vi "OdometricNavigation.vi"(0 "Wheel Angles (rad)":T3 {"RR Angle (rad)" scale=3.1416..-3.1416; "RL Angle (rad)" scale=3.1416..-3.1416; "FR Angle (rad)" scale=3.1416..-3.1416; "FL Angle (rad)" scale=3.1416..-3.1416}, 1 "Wheel Movements (in.)":cluster{"FL":dbl, "FR":dbl, "RL":dbl, "RR":dbl} {"RR" scale=-70.0..70.0; "RL" scale=-70.0..70.0; "FR" scale=-70.0..70.0; "FL" scale=-70.0..70.0}, 2 "Robot angle (degrees)":dbl(knob) scale=180.0..-180.0, 3 "x and y error minimum (in.)":dbl, 4 "error minimum for rotation (rad)":dbl) -> (17 "movement":cluster{"sy":dbl, "sx":dbl, "rot.":dbl})   [LabVIEW 2015, in "Team900SwerveDrive.lvlib"]
uses:
  Team900SwerveDrive.lvlib
  <vilib>/Analysis/baseanly.llb/Mean (DBL).vi
  SwerveGlobalData.vi
  <vilib>/Analysis/NI_AALBase.lvlib
panel:
  out "unhandled error data":dbl[][](array[numeric])
  out "Wheel X movements":T1
  out "Wheel Y movements":T2
  out "1-side error rotation (rad)":dbl
  out "compared":cluster{"sy":dbl, "sx":dbl, "rot.":dbl}[](array[cluster])
  out "Right Error":bool
  out "Front Error":bool
  out "Rear Error":bool
  out "Left Error":bool
  # "This VI should be run in periodic tasks at about 10 Hz, with the results being added to the\nX and Y elements of the 'Coordinates' variable from SwerveGlobalData.vi. Requires inputs of\ndelta(position) in inches and angle in radians for each wheel, as well as robot angle (in degrees)\nand error tolerances for the delta(position) and delta(angle) of the robot.\n\nThought: separate the X and Y coordinates of the robot and the heading of the robot into\ntwo separate global variables.\n\nThought: standardize degrees or radians throughout the code. Currently radians are used for\neverything except robot heading."
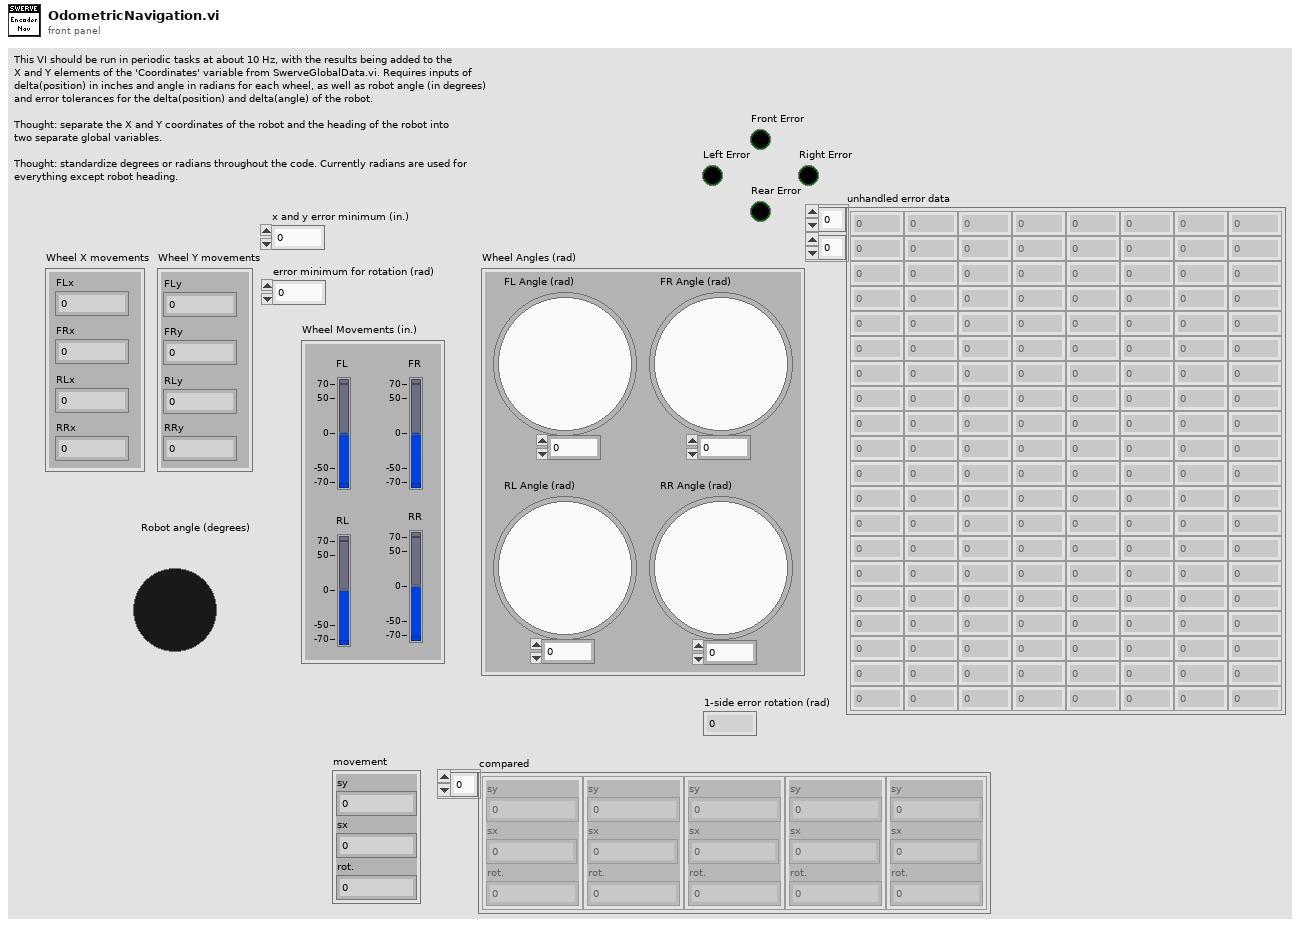
[diagram p1: front panel]
types:
  T1 = cluster{"FLx":dbl, "FRx":dbl, "RLx":dbl, "RRx":dbl}
  T2 = cluster{"FLy":dbl, "FRy":dbl, "RLy":dbl, "RRy":dbl}
  T3 = cluster{"FL Angle (rad)":dbl, "FR Angle (rad)":dbl, "RL Angle (rad)":dbl, "RR Angle (rad)":dbl}
  T4 = cluster{"[0]":dbl, "[1]":dbl, "[2]":dbl, "[3]":dbl}
  T5 = enum16{"no error", "front", "rear", "left", "right", "FL", "FR", "RL", "RR", "other"}
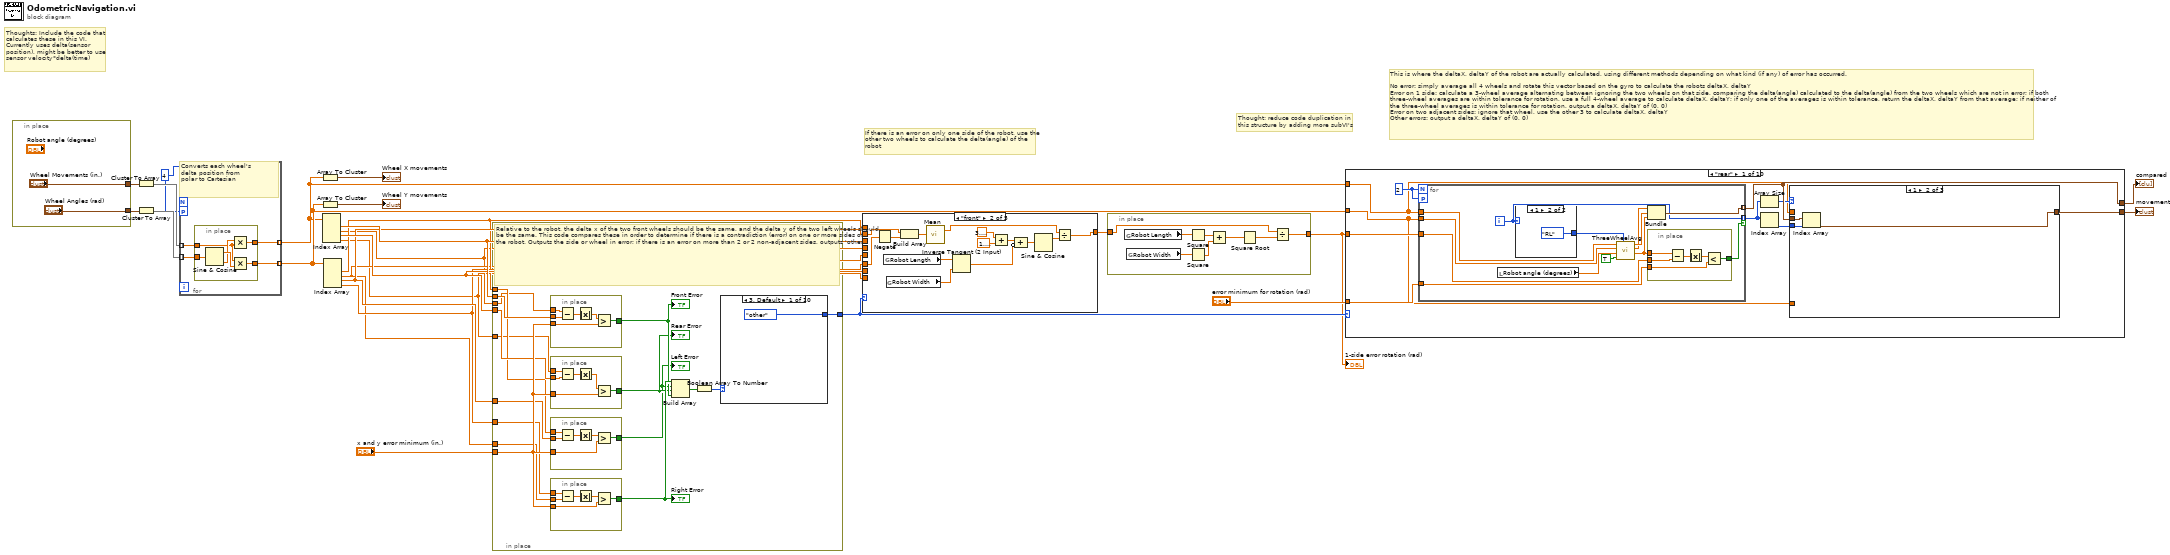
[diagram p0: block diagram]
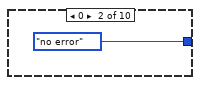
[diagram p2: hidden frame]
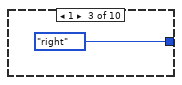
[diagram p3: hidden frame]
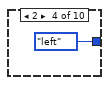
[diagram p4: hidden frame]
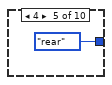
[diagram p5: hidden frame]
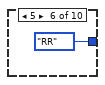
[diagram p6: hidden frame]
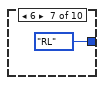
[diagram p7: hidden frame]
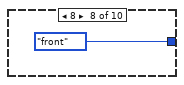
[diagram p8: hidden frame]
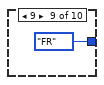
[diagram p9: hidden frame]
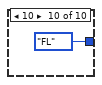
[diagram p10: hidden frame]
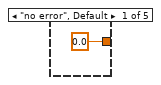
[diagram p11: hidden frame]
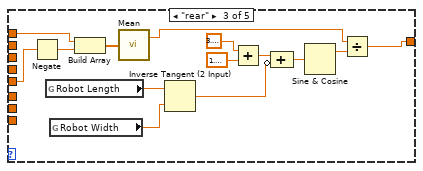
[diagram p12: hidden frame]
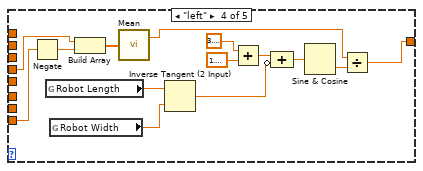
[diagram p13: hidden frame]
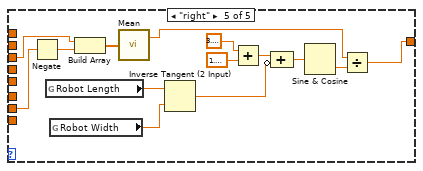
[diagram p14: hidden frame]
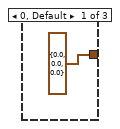
[diagram p15: hidden frame]
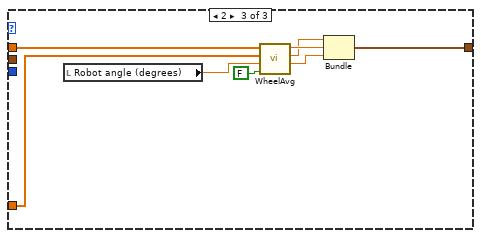
[diagram p16: hidden frame]
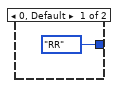
[diagram p17: hidden frame]
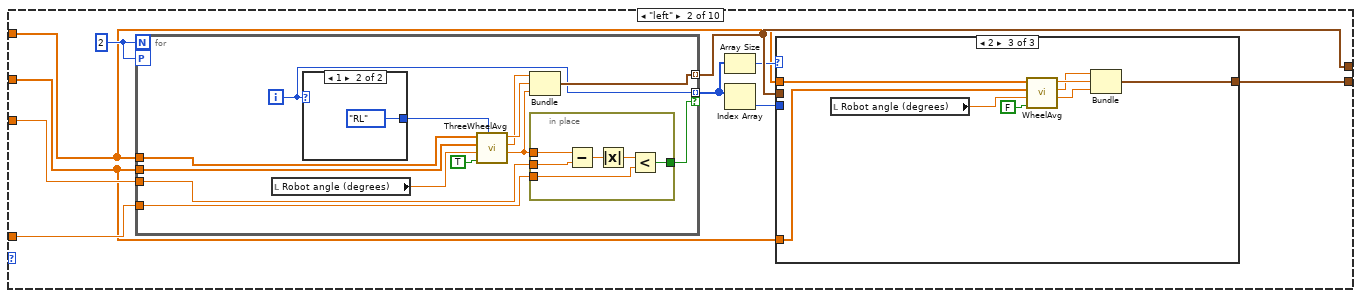
[diagram p18: hidden frame]
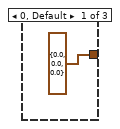
[diagram p19: hidden frame]
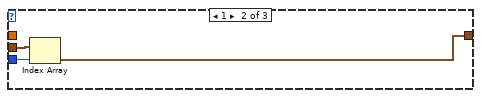
[diagram p20: hidden frame]
diagram:
  w16 = 4
  # "Thought: reduce code duplication in\nthis structure by adding more subVI's"
  # "This is where the deltaX, deltaY of the robot are actually calculated, using different methods depending on what kind (if any) of error has occurred.\n\nNo error: simply average all 4 wheels and rotate this vector based on the gyro to calculate the robots deltaX, deltaY\nError on 1 side: calculate a 3-wheel average alternating between ignoring the two wheels on that side, comparing the delta(angle) calculated to the delta(angle) from the two wheels which are not in error; if both \nthree-wheel averages are within tolerance for rotation, use a full 4-wheel average to calculate deltaX, deltaY; if only one of the averages is within tolerance, return the deltaX, deltaY from that average; if neither of\nthe three-wheel averages is within tolerance for rotation, output a deltaX, deltaY of (0, 0)\nError on two adjacent sides: ignore that wheel, use the other 3 to calculate deltaX, deltaY\nOther errors: output a deltaX, deltaY of (0, 0)"
  # "If there is an error on only one side of the robot, use the\nother two wheels to calculate the delta(angle) of the\nrobot"
  # "Thoughts: Include the code that\ncalculates these in this VI. \nCurrently uses delta(sensor\nposition), might be better to use\nsensor velocity*delta(time)"
  n1 = in-place {
    in-place-border: ["Wheel Movements (in.)"] -> w19
    in-place-border: ["Wheel Angles (rad)"] -> w18
  }
  n2 = Cluster To Array(cluster=w19) -> (array=w20:dbl[])
  n3 = Cluster To Array(cluster=w18) -> (array=w17:dbl[])
  n4 = for {
    N: w16 -> [_]
    tunnel: w20 -> [w30] mode=indexing
    tunnel: w17 -> [w29] mode=indexing
    workers-P: w16 -> [_]
    tunnel: [w28] -> w3 mode=indexing
    tunnel: [w27] -> w2 mode=indexing
    # "Converts each wheel's\ndelta position from\npolar to Cartesian"
    n5 = in-place {
      in-place-border: [w34] -> w27
      in-place-border: [w33] -> w28
      in-place-border: w30 -> [w32]
      in-place-border: w29 -> [w31]
      n6 = Sine & Cosine(0:w31) -> (1:w36:dbl, 2:w35:dbl)
      n7 = Multiply(x=w35, y=w32) -> (x*y=w34:dbl)
      n8 = Multiply(x=w32, y=w36) -> (x*y=w33:dbl)
    }
  }
  n9 = Array To Cluster(array=w2) -> (cluster=→"Wheel X movements":T4)
  n10 = Array To Cluster(array=w3) -> (cluster=→"Wheel Y movements":T4)
  n11 = Index Array(array=w2) -> (element #1=w12:dbl, element #2=w6:dbl, element #3=w11:dbl, element #4=w5:dbl)  [unwired: 4 in]
  n12 = Index Array(array=w3) -> (element #1=w8:dbl, element #2=w7:dbl, element #3=w10:dbl, element #4=w9:dbl)  [unwired: 4 in]
  n13 = in-place {
    in-place-border: "x and y error minimum (in.)" -> [w52]
    in-place-border: [w45] -> w13
    in-place-border: w12 -> [w44]
    in-place-border: w11 -> [w43]
    in-place-border: w10 -> [w42]
    in-place-border: w9 -> [w41]
    in-place-border: w8 -> [w40]
    in-place-border: w7 -> [w39]
    in-place-border: w6 -> [w38]
    in-place-border: w5 -> [w37]
    # "Relative to the robot, the delta x of the two front wheels should be the same, and the delta y of the two left wheels should be the same. This code compares these in order to determine if there is a contradiction (error) on one or more sides of the robot. Outputs the side or wheel in error; if there is an error on more than 2 or 2 non-adjacent sides, outputs 'other.'"
    n14 = in-place {
      in-place-border: [w66] -> w48
      in-place-border: w38 -> [w65]
      in-place-border: w44 -> [w64]
      in-place-border: w52 -> [w63]
      n15 = Subtract(x=w65, y=w64) -> (x-y=w68:dbl)
      n16 = Absolute Value(x=w68) -> (abs(x)=w67:dbl)
      n17 = Greater?(x=w67, y=w63) -> (0:w66:bool)
    }
    "Front Error" <- w48
    n18 = in-place {
      in-place-border: [w72] -> w47
      in-place-border: w37 -> [w71]
      in-place-border: w43 -> [w70]
      in-place-border: w52 -> [w69]
      n19 = Subtract(x=w71, y=w70) -> (x-y=w74:dbl)
      n20 = Absolute Value(x=w74) -> (abs(x)=w73:dbl)
      n21 = Greater?(x=w73, y=w69) -> (0:w72:bool)
    }
    "Rear Error" <- w47
    n22 = in-place {
      in-place-border: [w78] -> w46
      in-place-border: w40 -> [w77]
      in-place-border: w42 -> [w76]
      in-place-border: w52 -> [w75]
      n23 = Subtract(x=w77, y=w76) -> (x-y=w80:dbl)
      n24 = Absolute Value(x=w80) -> (abs(x)=w79:dbl)
      n25 = Greater?(x=w79, y=w75) -> (0:w78:bool)
    }
    "Left Error" <- w46
    n26 = in-place {
      in-place-border: [w84] -> w49
      in-place-border: w41 -> [w83]
      in-place-border: w39 -> [w82]
      in-place-border: w52 -> [w81]
      n27 = Subtract(x=w83, y=w82) -> (x-y=w86:dbl)
      n28 = Absolute Value(x=w86) -> (abs(x)=w85:dbl)
      n29 = Greater?(x=w85, y=w81) -> (0:w84:bool)
    }
    "Right Error" <- w49
    n30 = Build Array(w49, w46, w47, w48) -> (w51:bool[])
    n31 = Boolean Array To Number(Boolean array=w51) -> (number=w50:u32)
    n32 = case shown="3, Default" w50 {
      tunnel: [T5."other" T5."no error" T5."right" T5."left" T5."rear" T5."RR" T5."RL" T5."front" T5."FR" T5."FL"] -> w45
      frame 3, Default {
      }
      frame 0 {
      }
      frame 1 {
      }
      frame 2 {
      }
      frame 4 {
      }
      frame 5 {
      }
      frame 6 {
      }
      frame 8 {
      }
      frame 9 {
      }
      frame 10 {
      }
    }
  }
  n33 = case shown="\"front\"" w13 {
    tunnel: [0.0 w90 w102 w116 w132] -> w4
    tunnel: w12 -> [_ _ _ _ w131]
    tunnel: w11 -> [_ _ _ _ w130]
    tunnel: w10 -> [_ w89 _ _ _]
    tunnel: w9 -> [_ w88 _ _ _]
    tunnel: w8 -> [_ _ w105 _ _]
    tunnel: w7 -> [_ _ w104 _ _]
    tunnel: w6 -> [_ _ _ w118 _]
    tunnel: w5 -> [_ _ _ w117 _]
    frame "no error", Default {
    }
    frame "front" {
      n34 = Negate(x=w88) -> (-x=w100:dbl)
      n35 = global read "SwerveGlobalData.vi" "Robot Length"() -> (w93:dbl)
      n36 = global read "SwerveGlobalData.vi" "Robot Width"() -> (w94:dbl)
      n37 = Build Array(w89, w100) -> (w101:dbl[])
      n38 = call-poly <vilib>:"Mean.vi"("X"=w101) -> ("mean"=w99:dbl)  [unwired: 1 out]
      n39 = Inverse Tangent (2 Input)(1:w94, 2:w93) -> (0:w95:dbl)
      n40 = Add(x=3.141592653589793, y=1.5707963267948966) -> (x+y=w96:dbl)
      n41 = Compound Arithmetic op=ADD(w96, invert w95) -> (w92:dbl)
      n42 = Sine & Cosine(0:w92) -> (1:w91:dbl)  [unwired: 1 out]
      n43 = Divide(x=w99, y=w91) -> (x/y=w90:dbl)
    }
    frame "rear" {
      n44 = Negate(x=w104) -> (-x=w114:dbl)
      n45 = global read "SwerveGlobalData.vi" "Robot Length"() -> (w108:dbl)
      n46 = global read "SwerveGlobalData.vi" "Robot Width"() -> (w109:dbl)
      n47 = Build Array(w105, w114) -> (w115:dbl[])
      n48 = call-poly <vilib>:"Mean.vi"("X"=w115) -> ("mean"=w113:dbl)  [unwired: 1 out]
      n49 = Inverse Tangent (2 Input)(1:w109, 2:w108) -> (0:w103:dbl)
      n50 = Add(x=3.141592653589793, y=1.5707963267948966) -> (x+y=w110:dbl)
      n51 = Compound Arithmetic op=ADD(w110, invert w103) -> (w107:dbl)
      n52 = Sine & Cosine(0:w107) -> (1:w106:dbl)  [unwired: 1 out]
      n53 = Divide(x=w113, y=w106) -> (x/y=w102:dbl)
    }
    frame "left" {
      n54 = Negate(x=w117) -> (-x=w128:dbl)
      n55 = global read "SwerveGlobalData.vi" "Robot Length"() -> (w121:dbl)
      n56 = global read "SwerveGlobalData.vi" "Robot Width"() -> (w122:dbl)
      n57 = Build Array(w118, w128) -> (w129:dbl[])
      n58 = call-poly <vilib>:"Mean.vi"("X"=w129) -> ("mean"=w127:dbl)  [unwired: 1 out]
      n59 = Inverse Tangent (2 Input)(1:w122, 2:w121) -> (0:w123:dbl)
      n60 = Add(x=3.141592653589793, y=1.5707963267948966) -> (x+y=w124:dbl)
      n61 = Compound Arithmetic op=ADD(w124, invert w123) -> (w120:dbl)
      n62 = Sine & Cosine(0:w120) -> (2:w119:dbl)  [unwired: 1 out]
      n63 = Divide(x=w127, y=w119) -> (x/y=w116:dbl)
    }
    frame "right" {
      n64 = Negate(x=w130) -> (-x=w142:dbl)
      n65 = global read "SwerveGlobalData.vi" "Robot Length"() -> (w136:dbl)
      n66 = global read "SwerveGlobalData.vi" "Robot Width"() -> (w137:dbl)
      n67 = Build Array(w131, w142) -> (w143:dbl[])
      n68 = call-poly <vilib>:"Mean.vi"("X"=w143) -> ("mean"=w134:dbl)  [unwired: 1 out]
      n69 = Inverse Tangent (2 Input)(1:w137, 2:w136) -> (0:w138:dbl)
      n70 = Add(x=3.141592653589793, y=1.5707963267948966) -> (x+y=w139:dbl)
      n71 = Compound Arithmetic op=ADD(w139, invert w138) -> (w135:dbl)
      n72 = Sine & Cosine(0:w135) -> (2:w133:dbl)  [unwired: 1 out]
      n73 = Divide(x=w134, y=w133) -> (x/y=w132:dbl)
    }
  }
  n74 = in-place {
    in-place-border: w4 -> [w145]
    in-place-border: [w144] -> w1
    n75 = global read "SwerveGlobalData.vi" "Robot Length"() -> (w151:dbl)
    n76 = global read "SwerveGlobalData.vi" "Robot Width"() -> (w150:dbl)
    n77 = Square(x=w151) -> (x^2=w148:dbl)
    n78 = Square(x=w150) -> (x^2=w149:dbl)
    n79 = Add(x=w148, y=w149) -> (x+y=w147:dbl)
    n80 = Square Root(x=w147) -> (sqrt(x)=w146:dbl)
    n81 = Divide(x=w145, y=w146) -> (x/y=w144:dbl)
  }
  "1-side error rotation (rad)" <- w1
  n82 = case shown="\"rear\"" w13 {
    tunnel: [w157 w200 w243 w286 cluster{"mean":dbl, "mean":dbl, "mean":dbl}[] [] cluster{"mean":dbl, "mean":dbl, "mean":dbl}[] [] cluster{"mean":dbl, "mean":dbl, "mean":dbl}[] [] cluster{"mean":dbl, "mean":dbl, "mean":dbl}[] [] cluster{"mean":dbl, "mean":dbl, "mean":dbl}[] [] cluster{"mean":dbl, "mean":dbl, "mean":dbl}[] []] -> w23
    tunnel: "error minimum for rotation (rad)" -> [w161 w204 w247 w290 _ _ _ _ _ _]
    tunnel: [w158 w201 w244 w287 w333 w343 w353 w363 cluster{"mean":dbl, "mean":dbl, "mean":dbl} {"mean"=0.0, "mean"=0.0, "mean"=0.0} w379] -> w21
    tunnel: w3 -> [w153 w196 w239 w282 w329 w339 w349 w359 w368 w374]
    tunnel: w2 -> [w152 w195 w238 w281 w328 w338 w348 w358 w369 w373]
    tunnel: w1 -> [w156 w199 w242 w285 _ _ _ _ _ _]
    frame "rear" {
      w155 = 2
      n83 = for {
        N: w155 -> [_]
        tunnel: [w186] -> w157 mode=indexing
        tunnel: w161 -> [w185]
        tunnel: [w184] -> w160 mode=indexing if=w183
        tunnel: w153 -> [w180]
        tunnel: w152 -> [w179]
        tunnel: w156 -> [w174]
        workers-P: w155 -> [_]
        i -> [w184]
        n84 = local read "Robot angle (degrees)"() -> (w181:dbl)
        n85 = case shown="1" w184 {
          tunnel: [enum16{"FL", "FR", "RL", "RR"}."RR" ("Wheel Missing") enum16{"FL", "FR", "RL", "RR"}."RL" ("Wheel Missing")] -> w178
          frame 0, Default {
          }
          frame 1 {
          }
        }
        n86 = call "ThreeWheelAvg.vi"("Wheel Missing"=w178, "Calculate Rotation?"=TRUE, "Robot Angle (degrees)"=w181, "wheel Y movements (FL, FR, RL, RR)"=w180, "wheel X movements (FL, FR, RL, RR)"=w179) -> ("Rotation"=w175:dbl, "Y"=w176:dbl, "X"=w177:dbl)  [unwired: 4 in]
        n87 = Bundle("Y"=w176, "X"=w177, "Rotation"=w175) -> (w186:cluster{"Y":dbl, "X":dbl, "Rotation":dbl})  [unwired: 1 in]
        n88 = in-place {
          in-place-border: [w190] -> w183
          in-place-border: w185 -> [w189]
          in-place-border: w175 -> [w188]
          in-place-border: w174 -> [w187]
          n89 = Subtract(x=w188, y=w187) -> (x-y=w192:dbl)
          n90 = Absolute Value(x=w192) -> (abs(x)=w191:dbl)
          n91 = Less?(x=w191, y=w189) -> (x < y?=w190:bool)
        }
      }
      n92 = Array Size(array=w160) -> (size(s)=w154:i32)
      n93 = Index Array(array=w160) -> (element=w159:i32)  [unwired: 1 in]
      n94 = case shown="1" w154 {
        tunnel: w159 -> [_ w163 _]
        tunnel: [cluster{"Y":dbl, "X":dbl, "Rotation":dbl} {"Y"=0.0, "X"=0.0, "Rotation"=0.0} w165 w168] -> w158
        tunnel: w157 -> [_ w164 _]
        tunnel: w153 -> [_ _ w173]
        tunnel: w152 -> [_ _ w172]
        frame 0, Default {
        }
        frame 1 {
          n95 = Index Array(array=w164, index=w163) -> (element=w165:cluster{"Y":dbl, "X":dbl, "Rotation":dbl})
        }
        frame 2 {
          n96 = local read "Robot angle (degrees)"() -> (w166:dbl)
          n97 = call "WheelAvg.vi"("Calculate Rotation?"=FALSE, "Robot Angle (degrees)"=w166, "wheel Y movements (FL, FR, RL, RR)"=w173, "wheel X movements (FL, FR, RL, RR)"=w172) -> ("Rotation"=w169:dbl, "Y"=w170:dbl, "X"=w171:dbl)  [unwired: 5 in]
          n98 = Bundle("Y"=w170, "X"=w171, "Rotation"=w169) -> (w168:cluster{"Y":dbl, "X":dbl, "Rotation":dbl})  [unwired: 1 in]
        }
      }
    }
    frame "left" {
      w198 = 2
      n99 = for {
        N: w198 -> [_]
        tunnel: [w229] -> w200 mode=indexing
        tunnel: w204 -> [w228]
        tunnel: [w227] -> w203 mode=indexing if=w226
        tunnel: w196 -> [w223]
        tunnel: w195 -> [w222]
        tunnel: w199 -> [w217]
        workers-P: w198 -> [_]
        i -> [w227]
        n100 = local read "Robot angle (degrees)"() -> (w224:dbl)
        n101 = case shown="1" w227 {
          tunnel: [enum16{"FL", "FR", "RL", "RR"}."RR" ("Wheel Missing") enum16{"FL", "FR", "RL", "RR"}."RL" ("Wheel Missing")] -> w221
          frame 0, Default {
          }
          frame 1 {
          }
        }
        n102 = call "ThreeWheelAvg.vi"("Wheel Missing"=w221, "Calculate Rotation?"=TRUE, "Robot Angle (degrees)"=w224, "wheel Y movements (FL, FR, RL, RR)"=w223, "wheel X movements (FL, FR, RL, RR)"=w222) -> ("Rotation"=w218:dbl, "Y"=w219:dbl, "X"=w220:dbl)  [unwired: 4 in]
        n103 = Bundle("Y"=w219, "X"=w220, "Rotation"=w218) -> (w229:cluster{"Y":dbl, "X":dbl, "Rotation":dbl})  [unwired: 1 in]
        n104 = in-place {
          in-place-border: [w233] -> w226
          in-place-border: w228 -> [w232]
          in-place-border: w218 -> [w231]
          in-place-border: w217 -> [w230]
          n105 = Subtract(x=w231, y=w230) -> (x-y=w235:dbl)
          n106 = Absolute Value(x=w235) -> (abs(x)=w234:dbl)
          n107 = Less?(x=w234, y=w232) -> (x < y?=w233:bool)
        }
      }
      n108 = Array Size(array=w203) -> (size(s)=w197:i32)
      n109 = Index Array(array=w203) -> (element=w202:i32)  [unwired: 1 in]
      n110 = case shown="2" w197 {
        tunnel: w202 -> [_ w206 _]
        tunnel: [cluster{"Y":dbl, "X":dbl, "Rotation":dbl} {"Y"=0.0, "X"=0.0, "Rotation"=0.0} w208 w211] -> w201
        tunnel: w200 -> [_ w207 _]
        tunnel: w196 -> [_ _ w216]
        tunnel: w195 -> [_ _ w215]
        frame 0, Default {
        }
        frame 1 {
          n111 = Index Array(array=w207, index=w206) -> (element=w208:cluster{"Y":dbl, "X":dbl, "Rotation":dbl})
        }
        frame 2 {
          n112 = local read "Robot angle (degrees)"() -> (w209:dbl)
          n113 = call "WheelAvg.vi"("Calculate Rotation?"=FALSE, "Robot Angle (degrees)"=w209, "wheel Y movements (FL, FR, RL, RR)"=w216, "wheel X movements (FL, FR, RL, RR)"=w215) -> ("Rotation"=w212:dbl, "Y"=w213:dbl, "X"=w214:dbl)  [unwired: 5 in]
          n114 = Bundle("Y"=w213, "X"=w214, "Rotation"=w212) -> (w211:cluster{"Y":dbl, "X":dbl, "Rotation":dbl})  [unwired: 1 in]
        }
      }
    }
    frame "right" {
      w241 = 2
      n115 = for {
        N: w241 -> [_]
        tunnel: [w272] -> w243 mode=indexing
        tunnel: w247 -> [w271]
        tunnel: [w270] -> w246 mode=indexing if=w269
        tunnel: w239 -> [w266]
        tunnel: w238 -> [w265]
        tunnel: w242 -> [w260]
        workers-P: w241 -> [_]
        i -> [w270]
        n116 = local read "Robot angle (degrees)"() -> (w267:dbl)
        n117 = case shown="1" w270 {
          tunnel: [enum16{"FL", "FR", "RL", "RR"}."RR" ("Wheel Missing") enum16{"FL", "FR", "RL", "RR"}."RL" ("Wheel Missing")] -> w264
          frame 0, Default {
          }
          frame 1 {
          }
        }
        n118 = call "ThreeWheelAvg.vi"("Wheel Missing"=w264, "Calculate Rotation?"=TRUE, "Robot Angle (degrees)"=w267, "wheel Y movements (FL, FR, RL, RR)"=w266, "wheel X movements (FL, FR, RL, RR)"=w265) -> ("Rotation"=w261:dbl, "Y"=w262:dbl, "X"=w263:dbl)  [unwired: 4 in]
        n119 = Bundle("Y"=w262, "X"=w263, "Rotation"=w261) -> (w272:cluster{"Y":dbl, "X":dbl, "Rotation":dbl})  [unwired: 1 in]
        n120 = in-place {
          in-place-border: [w276] -> w269
          in-place-border: w271 -> [w275]
          in-place-border: w261 -> [w274]
          in-place-border: w260 -> [w273]
          n121 = Subtract(x=w274, y=w273) -> (x-y=w278:dbl)
          n122 = Absolute Value(x=w278) -> (abs(x)=w277:dbl)
          n123 = Less?(x=w277, y=w275) -> (x < y?=w276:bool)
        }
      }
      n124 = Array Size(array=w246) -> (size(s)=w240:i32)
      n125 = Index Array(array=w246) -> (element=w245:i32)  [unwired: 1 in]
      n126 = case shown="2" w240 {
        tunnel: w245 -> [_ w249 _]
        tunnel: [cluster{"Y":dbl, "X":dbl, "Rotation":dbl} {"Y"=0.0, "X"=0.0, "Rotation"=0.0} w251 w254] -> w244
        tunnel: w243 -> [_ w250 _]
        tunnel: w239 -> [_ _ w259]
        tunnel: w238 -> [_ _ w258]
        frame 0, Default {
        }
        frame 1 {
          n127 = Index Array(array=w250, index=w249) -> (element=w251:cluster{"Y":dbl, "X":dbl, "Rotation":dbl})
        }
        frame 2 {
          n128 = local read "Robot angle (degrees)"() -> (w252:dbl)
          n129 = call "WheelAvg.vi"("Calculate Rotation?"=FALSE, "Robot Angle (degrees)"=w252, "wheel Y movements (FL, FR, RL, RR)"=w259, "wheel X movements (FL, FR, RL, RR)"=w258) -> ("Rotation"=w255:dbl, "Y"=w256:dbl, "X"=w257:dbl)  [unwired: 5 in]
          n130 = Bundle("Y"=w256, "X"=w257, "Rotation"=w255) -> (w254:cluster{"Y":dbl, "X":dbl, "Rotation":dbl})  [unwired: 1 in]
        }
      }
    }
    frame "front" {
      w284 = 2
      n131 = for {
        N: w284 -> [_]
        tunnel: [w315] -> w286 mode=indexing
        tunnel: w290 -> [w314]
        tunnel: [w313] -> w289 mode=indexing if=w312
        tunnel: w282 -> [w309]
        tunnel: w281 -> [w308]
        tunnel: w285 -> [w303]
        workers-P: w284 -> [_]
        i -> [w313]
        n132 = local read "Robot angle (degrees)"() -> (w310:dbl)
        n133 = case shown="1" w313 {
          tunnel: [enum16{"FL", "FR", "RL", "RR"}."RR" ("Wheel Missing") enum16{"FL", "FR", "RL", "RR"}."RL" ("Wheel Missing")] -> w307
          frame 0, Default {
          }
          frame 1 {
          }
        }
        n134 = call "ThreeWheelAvg.vi"("Wheel Missing"=w307, "Calculate Rotation?"=TRUE, "Robot Angle (degrees)"=w310, "wheel Y movements (FL, FR, RL, RR)"=w309, "wheel X movements (FL, FR, RL, RR)"=w308) -> ("Rotation"=w304:dbl, "Y"=w305:dbl, "X"=w306:dbl)  [unwired: 4 in]
        n135 = Bundle("Y"=w305, "X"=w306, "Rotation"=w304) -> (w315:cluster{"Y":dbl, "X":dbl, "Rotation":dbl})  [unwired: 1 in]
        n136 = in-place {
          in-place-border: [w319] -> w312
          in-place-border: w314 -> [w318]
          in-place-border: w304 -> [w317]
          in-place-border: w303 -> [w316]
          n137 = Subtract(x=w317, y=w316) -> (x-y=w321:dbl)
          n138 = Absolute Value(x=w321) -> (abs(x)=w320:dbl)
          n139 = Less?(x=w320, y=w318) -> (x < y?=w319:bool)
        }
      }
      n140 = Array Size(array=w289) -> (size(s)=w283:i32)
      n141 = Index Array(array=w289) -> (element=w288:i32)  [unwired: 1 in]
      n142 = case shown="0, Default" w283 {
        tunnel: w288 -> [_ w292 _]
        tunnel: [cluster{"Y":dbl, "X":dbl, "Rotation":dbl} {"Y"=0.0, "X"=0.0, "Rotation"=0.0} w294 w297] -> w287
        tunnel: w286 -> [_ w293 _]
        tunnel: w282 -> [_ _ w302]
        tunnel: w281 -> [_ _ w301]
        frame 0, Default {
        }
        frame 1 {
          n143 = Index Array(array=w293, index=w292) -> (element=w294:cluster{"Y":dbl, "X":dbl, "Rotation":dbl})
        }
        frame 2 {
          n144 = local read "Robot angle (degrees)"() -> (w295:dbl)
          n145 = call "WheelAvg.vi"("Calculate Rotation?"=FALSE, "Robot Angle (degrees)"=w295, "wheel Y movements (FL, FR, RL, RR)"=w302, "wheel X movements (FL, FR, RL, RR)"=w301) -> ("Rotation"=w298:dbl, "Y"=w299:dbl, "X"=w300:dbl)  [unwired: 5 in]
          n146 = Bundle("Y"=w299, "X"=w300, "Rotation"=w298) -> (w297:cluster{"Y":dbl, "X":dbl, "Rotation":dbl})  [unwired: 1 in]
        }
      }
    }
    frame "FL" {
      # "fl"
      n147 = local read "Robot angle (degrees)"() -> (w331:dbl)
      n148 = call "ThreeWheelAvg.vi"("Wheel Missing"=enum16{"FL", "FR", "RL", "RR"}."FL", "Calculate Rotation?"=FALSE, "Robot Angle (degrees)"=w331, "wheel Y movements (FL, FR, RL, RR)"=w329, "wheel X movements (FL, FR, RL, RR)"=w328) -> ("Rotation"=w325:dbl, "Y"=w324:dbl, "X"=w326:dbl)  [unwired: 4 in]
      n149 = Bundle("Y"=w324, "X"=w326, "Rotation"=w325) -> (w333:cluster{"Y":dbl, "X":dbl, "Rotation":dbl})  [unwired: 1 in]
    }
    frame "FR" {
      # "fl"
      n150 = local read "Robot angle (degrees)"() -> (w341:dbl)
      n151 = call "ThreeWheelAvg.vi"("Wheel Missing"=enum16{"FL", "FR", "RL", "RR"}."FR", "Calculate Rotation?"=FALSE, "Robot Angle (degrees)"=w341, "wheel Y movements (FL, FR, RL, RR)"=w339, "wheel X movements (FL, FR, RL, RR)"=w338) -> ("Rotation"=w335:dbl, "Y"=w334:dbl, "X"=w336:dbl)  [unwired: 4 in]
      n152 = Bundle("Y"=w334, "X"=w336, "Rotation"=w335) -> (w343:cluster{"Y":dbl, "X":dbl, "Rotation":dbl})  [unwired: 1 in]
    }
    frame "RL" {
      # "fl"
      n153 = local read "Robot angle (degrees)"() -> (w351:dbl)
      n154 = call "ThreeWheelAvg.vi"("Wheel Missing"=enum16{"FL", "FR", "RL", "RR"}."RL", "Calculate Rotation?"=FALSE, "Robot Angle (degrees)"=w351, "wheel Y movements (FL, FR, RL, RR)"=w349, "wheel X movements (FL, FR, RL, RR)"=w348) -> ("Rotation"=w345:dbl, "Y"=w344:dbl, "X"=w346:dbl)  [unwired: 4 in]
      n155 = Bundle("Y"=w344, "X"=w346, "Rotation"=w345) -> (w353:cluster{"Y":dbl, "X":dbl, "Rotation":dbl})  [unwired: 1 in]
    }
    frame "RR" {
      # "fl"
      n156 = local read "Robot angle (degrees)"() -> (w361:dbl)
      n157 = call "ThreeWheelAvg.vi"("Wheel Missing"=enum16{"FL", "FR", "RL", "RR"}."RR", "Calculate Rotation?"=FALSE, "Robot Angle (degrees)"=w361, "wheel Y movements (FL, FR, RL, RR)"=w359, "wheel X movements (FL, FR, RL, RR)"=w358) -> ("Rotation"=w355:dbl, "Y"=w354:dbl, "X"=w356:dbl)  [unwired: 4 in]
      n158 = Bundle("Y"=w354, "X"=w356, "Rotation"=w355) -> (w363:cluster{"Y":dbl, "X":dbl, "Rotation":dbl})  [unwired: 1 in]
    }
    frame "other" {
      n159 = Build Array (concatenate)(w369, w368) -> (w367:dbl[])
      n160 = feedback #1(dbl[][] []) -> (w365:dbl[][])
      n161 = Build Array (concatenate)(w365, w367) -> (w366:dbl[][])
      "unhandled error data" <- w366
      n162 = feedback-in #1(w366) -> ()
    }
    frame "no error" {
      n163 = local read "Robot angle (degrees)"() -> (w372:dbl)
      n164 = call "WheelAvg.vi"("Calculate Rotation?"=FALSE, "Robot Angle (degrees)"=w372, "wheel Y movements (FL, FR, RL, RR)"=w374, "wheel X movements (FL, FR, RL, RR)"=w373) -> ("Rotation"=w376:dbl, "Y"=w377:dbl, "X"=w378:dbl)  [unwired: 5 in]
      n165 = Bundle("Y"=w377, "X"=w378, "Rotation"=w376) -> (w379:cluster{"Y":dbl, "X":dbl, "Rotation":dbl})  [unwired: 1 in]
    }
  }
  "compared" <- w23
  "movement" <- w21
